vi "Write I64 Direct Dispatch.vi"(8 "error in (no error)":errorcluster, 9 "Timeout (ms)":i32, 10 "Data":i64, 11 "CIFTag in":refnum<class "CIFChannels.lvclass">) -> (0 "error out":errorcluster, 1 "timed out?":bool, 3 "CIFTag out":refnum<class "CIF_NIChn_I64.lvclass">)   [LabVIEW 2021, in "CIF_NIChn_I64.lvclass"]
uses:
  CIF_NIChn_I64.lvclass
  CIF_NIChn_I64.lvclass/CIF_NIChn_I64.ctl
  e6e5dc56-0fe0-434b-816e-55c2e61471c2.vi
  NIChn/CIF_NIChn.lvclass
  D:/dev/Packages/Channel_Manager/src/CIF_NIChn/NIChn/CIF_NIChn.lvclass
  CIFChannels/CIFChannels.lvclass
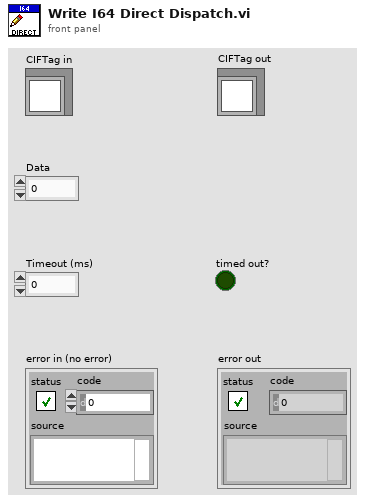
[diagram p1: front panel]
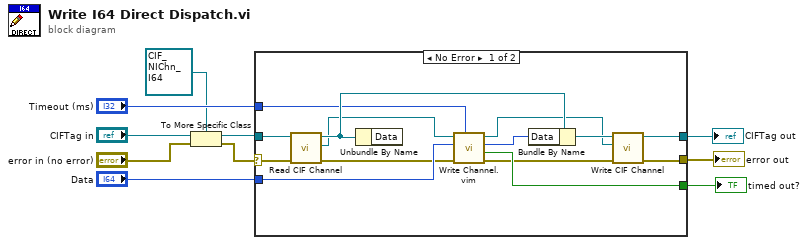
[diagram p0: block diagram]
diagram:
  n1 = To More Specific Class(target class=refnum<class "CIF_NIChn_I64.lvclass"> refnum ("CIFTag in"), reference="CIFTag in", error in="error in (no error)") -> (specific class reference=w3:refnum<class "CIF_NIChn_I64.lvclass">, error out=w1:errorcluster)
  n2 = case shown="No Error" w1 {
    selector: w1 -> [w21 w26]
    tunnel: [w15 w26] -> w10
    tunnel: [w17 w25] -> w9
    tunnel: w3 -> [w22 w25]
    tunnel: "Data" -> [w24 _]
    tunnel: [w23 _] -> w7
    tunnel: "Timeout (ms)" -> [w12 _]
    frame No Error {
      n3 = call "Read CIF Channel.vi"("error in (no error)"=w21, "CIFTag in"=w22) -> ("error out"=w19:errorcluster, "CIF Channel"=w14:refnum<k21>, "CIFTag out"=w20:refnum<class "CIF_NIChn_I64.lvclass">)  [unwired: 7 in]
      n4 = Unbundle By Name(w20) -> ()  [unwired: 1 out]
      n5 = call "Write Channel.vim"("Timeout (ms)"=w12, "error in"=w19, "Data in"=w24, "CIF Channel in"=w14) -> ("error out"=w16:errorcluster, "Timed out?"=w23:bool, "Data out"=w11:i64, "CIF Channel out"=w13:refnum<k21>)  [unwired: 4 in]
      n6 = Bundle By Name(cluster=w20, "Data"=w11) -> (w18:refnum<class "CIF_NIChn_I64.lvclass">)
      n7 = call "Write CIF Channel.vi"("error in (no error)"=w16, "CIF Channel"=w13, "CIFTag in"=w18) -> ("error out"=w15:errorcluster, "CIFTag out"=w17:refnum<class "CIF_NIChn_I64.lvclass">)  [unwired: 7 in]
    }
    frame Error {
    }
  }
  "error out" <- w10
  "CIFTag out" <- w9
  "timed out?" <- w7
